vi "Warmup Saving.vi"(8 "connection information":path, 9 "TimeMeasured":string[](array[string]), 10 "DC_SN":string, 11 "Frequency":string[](array[string])) -> ()   [LabVIEW 2024]
uses:
  <vilib>/addons/database/NI_Database_API.lvlib
  <vilib>/addons/database/_DB Variant To Data/Database Variant To Data.xnode
  <vilib>/addons/database/Connection.llb/Conn Execute.vi
  <vilib>/addons/database/Connection.llb/DB Tools Open Connec (Path).vi
  <vilib>/addons/database/Recordset.llb/Rec Destroy - Connection.vi
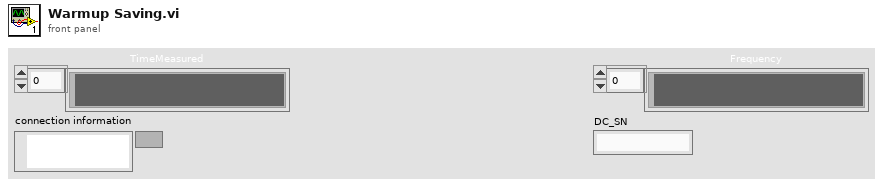
[diagram p1: front panel]
types:
  T1 = typedef "NI_Database_API.lvlib/Conn ObjectReference.ctl" = refnum<k1>
  T2 = typedef "NI_Database_API.lvlib/Rec ObjectReference.ctl" = refnum<k1>
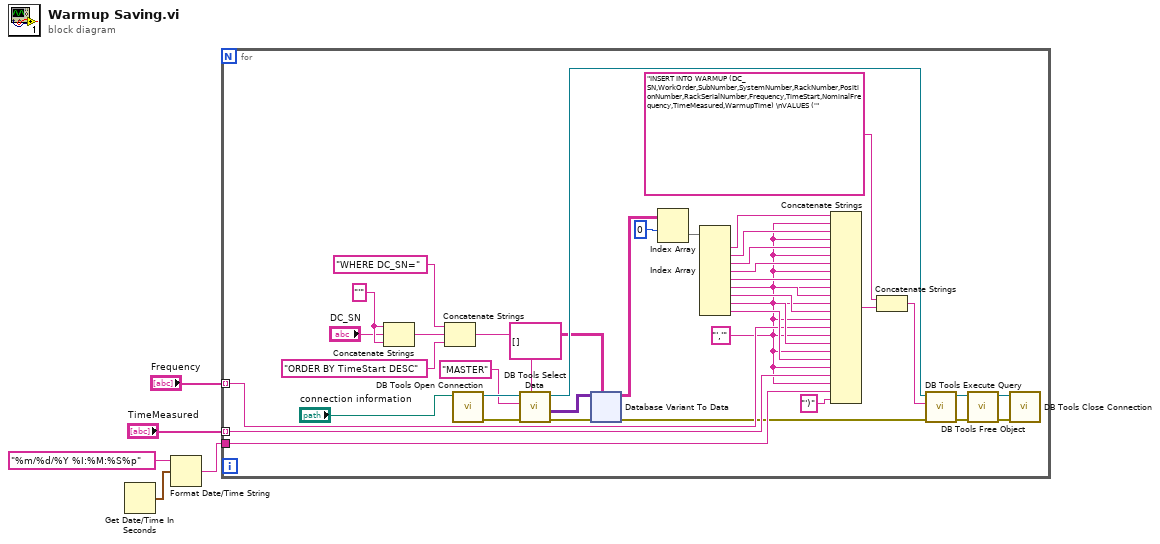
[diagram p0: block diagram]
diagram:
  n1 = Get Date/Time In Seconds() -> (seconds since 1Jan1904=w3:timestamp)
  n2 = Format Date/Time String(time format string (%c)="%m/%d/%Y %I:%M:%S%p", seconds (now)=w3) -> (date/time string=w1:string)  [unwired: 1 in]
  n3 = for {
    tunnel: "Frequency" -> [w27] mode=indexing
    tunnel: "TimeMeasured" -> [w25] mode=indexing
    tunnel: w1 -> [w22]
    w29 = "'" ("string")
    w23 = "','"
    n4 = Concatenate Strings(w29, "DC_SN", w29) -> (w28:string)
    n5 = Concatenate Strings("WHERE DC_SN=" ("SQL Query"), w28, "ORDER BY TimeStart DESC" ("string")) -> (w8:string)
    n6 = call-poly <vilib>:"DB Tools Open Connection.vi"("connection information"="connection information") -> ("error out"=w17:errorcluster, "connection reference"=w16:T1)  [unwired: 7 in]
    n7 = call <vilib>:"DB Tools Select Data.vi"("condition"=w8, "error in (no error)"=w17, "table"="MASTER", "connection reference"=w16) -> ("error out"=w19:errorcluster, "data"=w18:variant[][], "connection reference out"=w15:T1)  [unwired: 2 in]
    n8 = xnode "Database Variant To Data"("database variant"=w18, "error in (no error)"=w19, "type"=string[][] []) -> ("data"=w6:string[][], "error out"=w20:errorcluster)
    n9 = Index Array(array=w6, index (row)=0 ("disabled index (row)")) -> (element=w42:string[])  [unwired: 1 in]
    n10 = Index Array(array=w42) -> (element #1=w40:string, element #2=w39:string, element #3=w38:string, element #4=w37:string, element #5=w31:string, element #6=w30:string, element #7=w34:string, element #8=w44:string, element #9=w32:string)  [unwired: 9 in]
    n11 = Concatenate Strings(w40, w23, w39, w23, w38, w23, w37, w23, w31, w23, w30, w23, w34, w23, w27, w23, w44, w23, w32, w23, w25, w23, w22, "')" ("string")) -> (w41:string)
    n12 = Concatenate Strings("INSERT INTO WARMUP (DC_SN,WorkOrder,SubNumber,SystemNumber,RackNumber,PositionNumber,RackSerialNumber,Frequency,TimeStart,NominalFrequency,TimeMeasured,WarmupTime) \nVALUES ('" ("string"), w41) -> (w7:string)
    n13 = call-poly <vilib>:"DB Tools Execute Query.vi"("error in (no error)"=w20, "SQL query"=w7, "connection reference"=w15) -> ("error out"=w12:errorcluster, "recordset reference"=w11:T2)  [unwired: 5 in]
    n14 = call-poly <vilib>:"DB Tools Free Object.vi"("error in (no error)"=w12, "recordset reference"=w11) -> ("error out"=w14:errorcluster, "connection reference"=w13:T1)  [unwired: 8 in]
    n15 = call <vilib>:"DB Tools Close Connection.vi"("error in (no error)"=w14, "connection reference"=w13) -> ()  [unwired: 5 in, 1 out]
  }
